vi "PRAT Update Status Color.vi"(6 "Disable Cycle Counter":bool, 8 "Error In":errorcluster, 9 "Disable Station":T3, 10 "Draw Station is Drawing Water":bool, 11 "Display Data (RLT) In":T1 {"Current Display" format="%.2f"; "Cycle Count Display" format="%04d"}) -> (0 "Error Out":errorcluster, 3 "Display Data (RLT) Out":T1 {"Current Display" format="%.2f"; "Cycle Count Display" format="%04d"})   [LabVIEW 2019]
uses:
  Type Definitions/HEWH RLT Station Disable.ctl
  Utility/Save File/Public/Type Definitions/Save File Appliance Display.ctl
  Utility/Save File/Public/Type Definitions/Save File Unit Type.ctl
  Utility/Save File/Global/Save File Globals HCC.vi
  Utility/Save File/Save File.lvlib
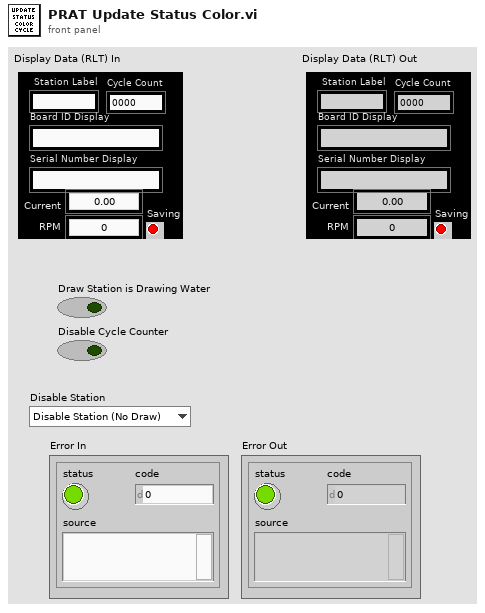
[diagram p1: front panel]
types:
  T1 = typedef "Save File Appliance Display.ctl" = cluster{"Status Color":u32, "Serial Number Display":string, "Cycle Count Display":i32, "Station Label Display":string, "Current Run Start Time Display":dbl, "Board ID Display":string, "RPM Display":u32, "Current Display":dbl, "Current Path Display":path, "Saving Display":bool, "Unit Type Display":T2, "Total Time On Display":dbl, "UI Button":bool}
  T2 = typedef "Save File.lvlib/Save File Unit Type.ctl" = enum32{"", "Viper", "Hawk", "2015"}
  T3 = typedef "HEWH RLT Station Disable.ctl" = enum16{"Disable Station (No Draw)", "Enable Station"}
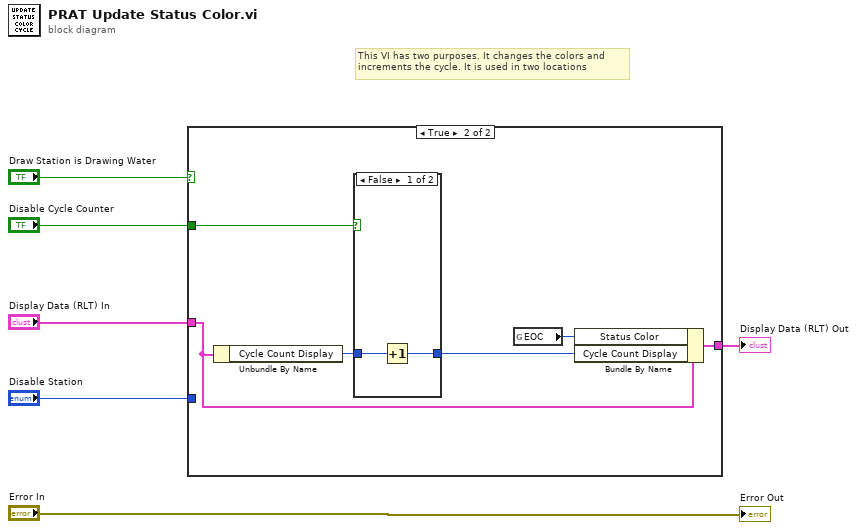
[diagram p0: block diagram]
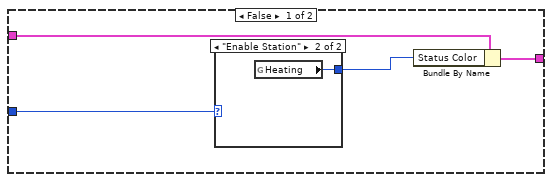
[diagram p2: hidden frame]
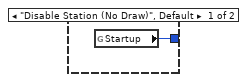
[diagram p3: hidden frame]
diagram:
  # "This VI has two purposes. It changes the colors and \nincrements the cycle. It is used in two locations"
  n1 = case shown="True" "Draw Station is Drawing Water" {
    tunnel: "Disable Station" -> [w10 _]
    tunnel: "Display Data (RLT) In" -> [w7 w16]
    tunnel: [w8 w18] -> w1
    tunnel: "Disable Cycle Counter" -> [_ w13]
    frame False {
      n2 = case shown="\"Enable Station\"" w10 {
        tunnel: [w11 w12] -> w9
        frame "Disable Station (No Draw)", Default {
          n3 = global read "Save File Globals HCC.vi" "Startup"() -> (w11:u32)
        }
        frame "Enable Station" {
          n4 = global read "Save File Globals HCC.vi" "Heating"() -> (w12:u32)
        }
      }
      n5 = Bundle By Name(cluster=w7, "Status Color"=w9) -> (w8:T1)
    }
    frame True {
      n6 = Unbundle By Name(w16) -> ("Cycle Count Display"=w15:i32)
      n7 = case shown="False" w13 {
        tunnel: w15 -> [w20 w21]
        tunnel: [w19 w21] -> w14
        frame False {
          n8 = Increment(x=w20) -> (x+1=w19:i32)
        }
        frame True {
        }
      }
      n9 = global read "Save File Globals HCC.vi" "EOC"() -> (w17:u32)
      n10 = Bundle By Name(cluster=w16, "Status Color"=w17, "Cycle Count Display"=w14) -> (w18:T1)
    }
  }
  "Display Data (RLT) Out" <- w1
  "Error Out" <- "Error In"
